vi "AutoDriveTo.vi"(9 "EndAngle":dbl, 10 "EndCoordinates":dbl[](array[numeric]), 11 "Coordinates":dbl[](array[numeric])) -> (3 "ThereYet?":bool)   [LabVIEW 2018]
uses:
  Globals.vi
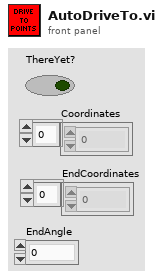
[diagram p1: front panel]
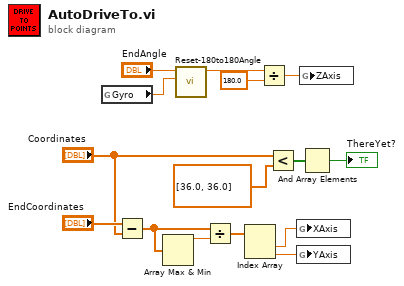
[diagram p0: block diagram]
diagram:
  n1 = global read "Globals.vi" "Gyro"() -> (w4:dbl)
  n2 = Subtract(x="EndCoordinates", y="Coordinates") -> (x-y=w15:dbl[])
  n3 = Array Max & Min(array=w15) -> (max value=w14:dbl)  [unwired: 3 out]
  n4 = call "Reset-180to180Angle.vi"("Offset"=w4, "AngleInput"="EndAngle") -> ("AngleOutput"=w3:dbl)  [unwired: 9 in]
  n5 = Divide(x=w15, y=w14) -> (x/y=w13:dbl[])
  n6 = Index Array(array=w13) -> (element #1=w12:dbl, element #2=w11:dbl)  [unwired: 2 in]
  n7 = Divide(x=w3, y=180.0) -> (x/y=w1:dbl)
  n8 = Less?(x="Coordinates", y=dbl[] [36.0, 36.0]) -> (x < y?=w9:bool[])
  n9 = global write "Globals.vi" "XAxis"(w12) -> ()
  n10 = global write "Globals.vi" "YAxis"(w11) -> ()
  n11 = global write "Globals.vi" "ZAxis"(w1) -> ()
  n12 = And Array Elements(Boolean array=w9) -> (logical AND=→"ThereYet?":bool)
